vi "HOST_timesharelargearraywithdatacollection_2-27-23.vi"() -> ()   [LabVIEW 2020]
uses:
  <vilib>/rvi/interface/nirviMethod/nirviMethod.xnode
  <vilib>/rvi/errors/niLvFpgaMergeErrorWithErrorCode.vi
  <instrlib>/_niInstr/Streaming/v1/Host/niInstr Streaming v1 Host.lvlib
  <vilib>/rvi/interface/nirviReadWriteControl/nirviReadWriteControl.xnode
  <vilib>/rvi/interface/nirviCloseFPGA/nirviCloseFPGA.xnode
  <vilib>/rvi/interface/nirviOpenFPGA/nirviOpenFPGA.xnode
  <vilib>/rvi/interface/Simulation/niFpgaSimulationCallBeginRW.vi
  <vilib>/rvi/errors/niLvFpgaAdjustHostInterfaceError.vi
  NiFpgaLv.dll
  <vilib>/Utility/error.llb/Error Cluster From Error Code.vi
  <vilib>/Utility/file.llb/Write Delimited Spreadsheet (string).vi
  FPGA Bitfiles/rfsignal_FPGATarget_timesharelargear_57WzZEcFPMM.lvbitx
  <vilib>/FPGAPlugInAG/PXIe-7972R/niLvFpga_Open_PXIe-7972R.vi
  <vilib>/rvi/interface/common/dynamic/niFpgaDynamicAddResources.vi
  <vilib>/FPGAPlugInAG/Dynamic/niLvFpga_ConfigureFifo_Dynamic.vi
  <vilib>/FPGAPlugInAG/Dynamic/niLvFpga_StartFifo_Dynamic.vi
  <vilib>/FPGAPlugInAG/Dynamic/niLvFpga_WriteFifo_Dynamic.vi
  <vilib>/FPGAPlugInAG/Dynamic/niLvFpga_Close_Dynamic.vi
  <instrlib>/_niInstr/Streaming/v1/Host/Public/Start Continuous Stream.vi
  <instrlib>/_niInstr/Streaming/v1/Host/Public/Wait for Stream.vi
  <instrlib>/_niInstr/Streaming/v1/Host/Public/Start Finite Stream.vi
  <vilib>/FPGAPlugInAG/Dynamic/niLvFpga_ReadFifo_Dynamic.vi
  <vilib>/userDefined/Silver/nirio_resource_slv.ctl
  Controls/Clock Select.ctl
panel:
  in  "Data Trigger Level (V)":dbl
  in  "Record Size":u16=1024
  out "AI":waveform(dbl)[](graph)
  in  "Data Trigger When":enum8{"Trigger Above", "Trigger Below"}(ring)
  in  "Trigger Type":enum8{"Immediate", "Data Trigger", "TRIG input"}(ring)
  in  "Burst Power":bool
  in  "Correct Gains":bool
  in  "% of max CH 0":dbl=100.0
  in  "% of max CH 1":dbl=100.0
  in  "CH 1 Number of Waves":i8=1
  in  "write time ch0":bool
  in  "Record time for power sweep CH0":bool
  in  "Record time for power sweep CH1":bool
  in  "write time ch1":bool
  in  "save path for power calibration (dialog if empty)":path=path "D:/Lab Data/20220720/frequencysweep/CH0sweep-5to5.txt"
  out "time check":u16=1
  in  "Cycles per step":u16=30
  in  "Gain Scan Endpoint (CH1)":dbl[](array[numeric])=[0.0, 100.0, 100.0, 100.0, 100.0, 100.0, 100.0, 100.0, 100.0, 100.0]
  in  "Gain Scan Endpoint (CH0)":dbl[](array[numeric])=[100.0, 100.0, 100.0, 100.0, 100.0, 100.0, 100.0, 100.0, 100.0, 100.0, 100.0, 100.0, 100.0, 100.0, 100.0, 100.0, 100.0, 100.0, 100.0, 100.0, 100.0, 100.0, 100.0, 100.0, 100.0, 100.0, 100.0, 100.0, 100.0, 100.0, 100.0]
  in  "Scan End Setpoint (CH1)":dbl[](array[numeric])=[0.0, 1.0, 0.0, 0.0, 0.0, 0.0, 0.0, 0.0, 0.0, 0.0, 0.0, 0.0, 0.0, 0.0, 0.0, 0.0, 0.0, 0.0, 0.0, 0.0, 0.0, 0.0, 0.0, 0.0, 0.0, 0.0, 0.0, 0.0, 0.0, 0.0, 0.0] format="%#_10f"
  in  "Scan CH1":bool
  in  "Scan CH0":bool
  in  "Fq Scan Endpoint (CH0)":dbl[](array[numeric])=[0.0, 0.0, 0.0, 0.0, 0.0, 0.0, 0.0, 0.0, 0.0, 0.0, 0.0, 0.0, 0.0, 0.0, 0.0, 0.0, 0.0, 0.0, 0.0, 0.0, 0.0, 0.0, 0.0, 0.0, 0.0, 0.0, 0.0, 0.0, 0.0, 0.0, 0.0, 0.0, 0.0, 0.0, 0.0] format="%#_10f"
  in  "Amp mod on/off":bool[](array[boolean])=[FALSE, FALSE, FALSE, FALSE, FALSE, FALSE, FALSE, FALSE, FALSE, FALSE]
  in  "Mod Amp (%)":fxp<+,16,1>[](array[numeric])=[1.0, 1.0, 1.0, 1.0, 1.0, 1.0, 1.0, 1.0, 1.0, 1.0]
  in  "Mod Fq (Hz) 3":dbl[](array[numeric])=[1.0, 1.0, 1.0, 1.0, 1.0, 1.0, 1.0, 1.0, 1.0, 1.0] format="%#5.5f"
  in  "Wave 2 mod on/off":bool[](array[boolean])=[FALSE, FALSE, FALSE, FALSE, FALSE, FALSE, FALSE, FALSE, FALSE, FALSE]
  in  "Mod strength (Hz) 2":dbl[](array[numeric])=[100000.0, 100000.0, 100000.0, 100000.0, 100000.0, 100000.0, 100000.0, 100000.0, 100000.0, 100000.0] format="%#_6p"
  in  "Mod Fq (Hz) 2":dbl[](array[numeric])=[1.0, 1.0, 1.0, 1.0, 1.0, 1.0, 1.0, 1.0, 1.0, 1.0] format="%#5.5f"
  in  "Wave 1 mod on/off":bool[](array[boolean])=[FALSE, FALSE, FALSE, FALSE, FALSE, FALSE, FALSE, FALSE, FALSE, FALSE]
  in  "Mod strength (Hz)":dbl[](array[numeric])=[100000.0, 100000.0, 100000.0, 100000.0, 100000.0, 100000.0, 100000.0, 100000.0, 100000.0, 100000.0] format="%#_6p"
  in  "Mod Time (Hz)":dbl[](array[numeric])=[1.0, 1.0, 1.0, 1.0, 1.0, 1.0, 1.0, 1.0, 1.0, 1.0] format="%#5.5p"
  in  "Gain Scan Step Size % (CH1)":dbl=0.5
  in  "Gain Scan Step Size % (CH0)":dbl=0.1
  in  "Fq Scan Step Size MHz (CH1)":dbl=0.09999999999999999
  in  "Fq Scan Step Size MHz (CH0)":dbl=0.09999999999999999
  in  "CH 0 Number of Waves":i8=1
  in  "Wave Reader CH 1 (X)":dbl[](array[numeric])=[0.0, 1.0, 0.0, 0.0, 0.0, 0.0, 0.0, 0.0, 0.0, 0.0, 0.0, 0.0, 0.0, 0.0, 0.0, 0.0, 0.0, 0.0, 0.0, 0.0, 0.0, 0.0, 0.0, 0.0, 0.0, 0.0, 0.0, 0.0, 0.0, 0.0, 0.0] format="%#_15f"
  in  "Gain CH 1 (%)":dbl[](array[numeric])=[100.0, 0.0, 0.0, 0.0, 0.0, 0.0, 0.0, 0.0, 0.0, 0.0]
  in  "Remove transition edges":i32=5
  in  "Time per beam in us":i32=20
  in  "stop":bool
  in  "Gain CH 0 (%)":dbl[](array[numeric])=[100.0, 100.0, 100.0, 100.0, 100.0, 100.0, 100.0, 100.0, 100.0, 100.0, 100.0, 100.0, 100.0, 100.0, 100.0, 100.0, 100.0, 100.0, 100.0, 100.0, 100.0, 100.0, 100.0, 100.0, 100.0, 100.0, 100.0, 100.0, 100.0, 100.0, 100.0]
  in  "Wave Reader CH 0 (MHz from center)":dbl[](array[numeric])=[0.0, 0.0, 0.0, 0.0, 0.0, 0.0, 0.0, 0.0, 0.0, 0.0, 0.0, 0.0, 0.0, 0.0, 0.0, 0.0, 0.0, 0.0, 0.0, 0.0, 0.0, 0.0, 0.0, 0.0, 0.0, 0.0, 0.0, 0.0, 0.0, 0.0, 0.0, 0.0, 0.0, 0.0, 0.0] format="%#_13f"
  in  "Magnitude Initialization Vpp":dbl[](array[numeric])=[1.0, 1.0] format="%0.2p"
  in  "Frequencies (Hz)":dbl[](array[numeric])=[10000.0, 10000.0] format="%5.0p"
  in  "Signal Type":T1(ring)
  in  "Sampling Info":cluster{"Fs":dbl, "#s":dbl}={"Fs"=163840000.0, "#s"=65536.0} {"Fs" format="%#_5p"}
  out "Error Out":errorcluster
  in  "Update Waveform":bool
  in  "AO Channel":T2(ring)
  in  "Clock Select":T3 items=["Internal Clock", "Internal Clock w/ Ref via CLK/REF IN", "Internal Clock w/ Ref via Sync Clock", "External Clock via CLK/REF IN"]
  in  "Rate of External Sample Clock (MHz)":u16=100 min=60 max=100 step=1
  in  "RIO Resource":T4="RIO1"
  # "General Feedback Settings"
  # "Time cycle loop processing"
  # "Shared Feedback Controls"
  # "Don't change"
  # "Modulates the output frequencies of CH 1 in a sine wave pattern\n\nMod time: Sets how fast the modulation goes\n     (e.g. 1 Hz means it will go through a full cycle in 1 second)\n\nMod strength: Sets the amplitude of the modulation\n     (e.g. 100kHz means that the frequency will go between \n      set frequency + 100kHz and set frequency - 100kHz)"
  # "Modulates the output frequencies of CH 0 in a sine wave pattern\n\nMod time: Sets how fast the modulation goes\n     (e.g. 1 Hz means it will go through a full cycle in 1 second)\n\nMod strength: Sets the amplitude of the modulation\n     (e.g. 100kHz means that the frequency will go between \n      set frequency + 100kHz and set frequency - 100kHz)"
  # "Modulates the output amplitude of CH 0 in a sine wave pattern\n\nMod time: Sets how fast the modulation goes\n     (e.g. 1 Hz means it will go through a full cycle in 1 second)\n\nMod strength: Sets the amplitude of the modulation\n     (e.g. 5% means that the amplitude will go between \n      set amp + 5%  and set amp  - 5%)"
  # "Waveform Initialization"
  # "These allow you to smoothly ramp between frequencies or gain settings for each individual beam.\nThe channels scan independently, but it will simultaneously ramp every fq/gain in the channel to their desired point.\nThey should update to match the main control setting when scanning is not enabled."
  # "DO NOT CHANGE"
  # "Main control for the tones played on FPGA analog out 0\nSets the base, static frequency to play\n\nIt will play the first n rows of tones, \nwhere n is the \"# of beams\" value."
  # "Main control for the tones played on FPGA analog out 1\nSets the base, static frequency to play"
  # "Do not change these values while waiting for scan"
  # "Ch 0 Wave Sin Modulation"
  # "Ch 1 Wave Sin Modulation"
  # "Amplitude Sin Modulation"
  # "Ch 0 Output Waveforms"
  # "Ch 1 Output Waveforms"
  # "Ch0"
  # "Ch1"
  # "Controls the Output of the FPGA\nEach row corresponds to one beam created by the AOD\nCH 0 is Output 0 on the FPGA card and controls the () direction on the AOD; CH 1 is Output 1 on the FPGA card and controls the () direction on the AOD\n\n0 means that the center frequency (27MHz) is output. The total range is +-8MHz, but there too much efficiency loss after 4 MHz away from the center frequency\n\nThe gain is the percentage of the 1Vpp initialized voltage to output. It is in percentage and goes from 0 - 100"
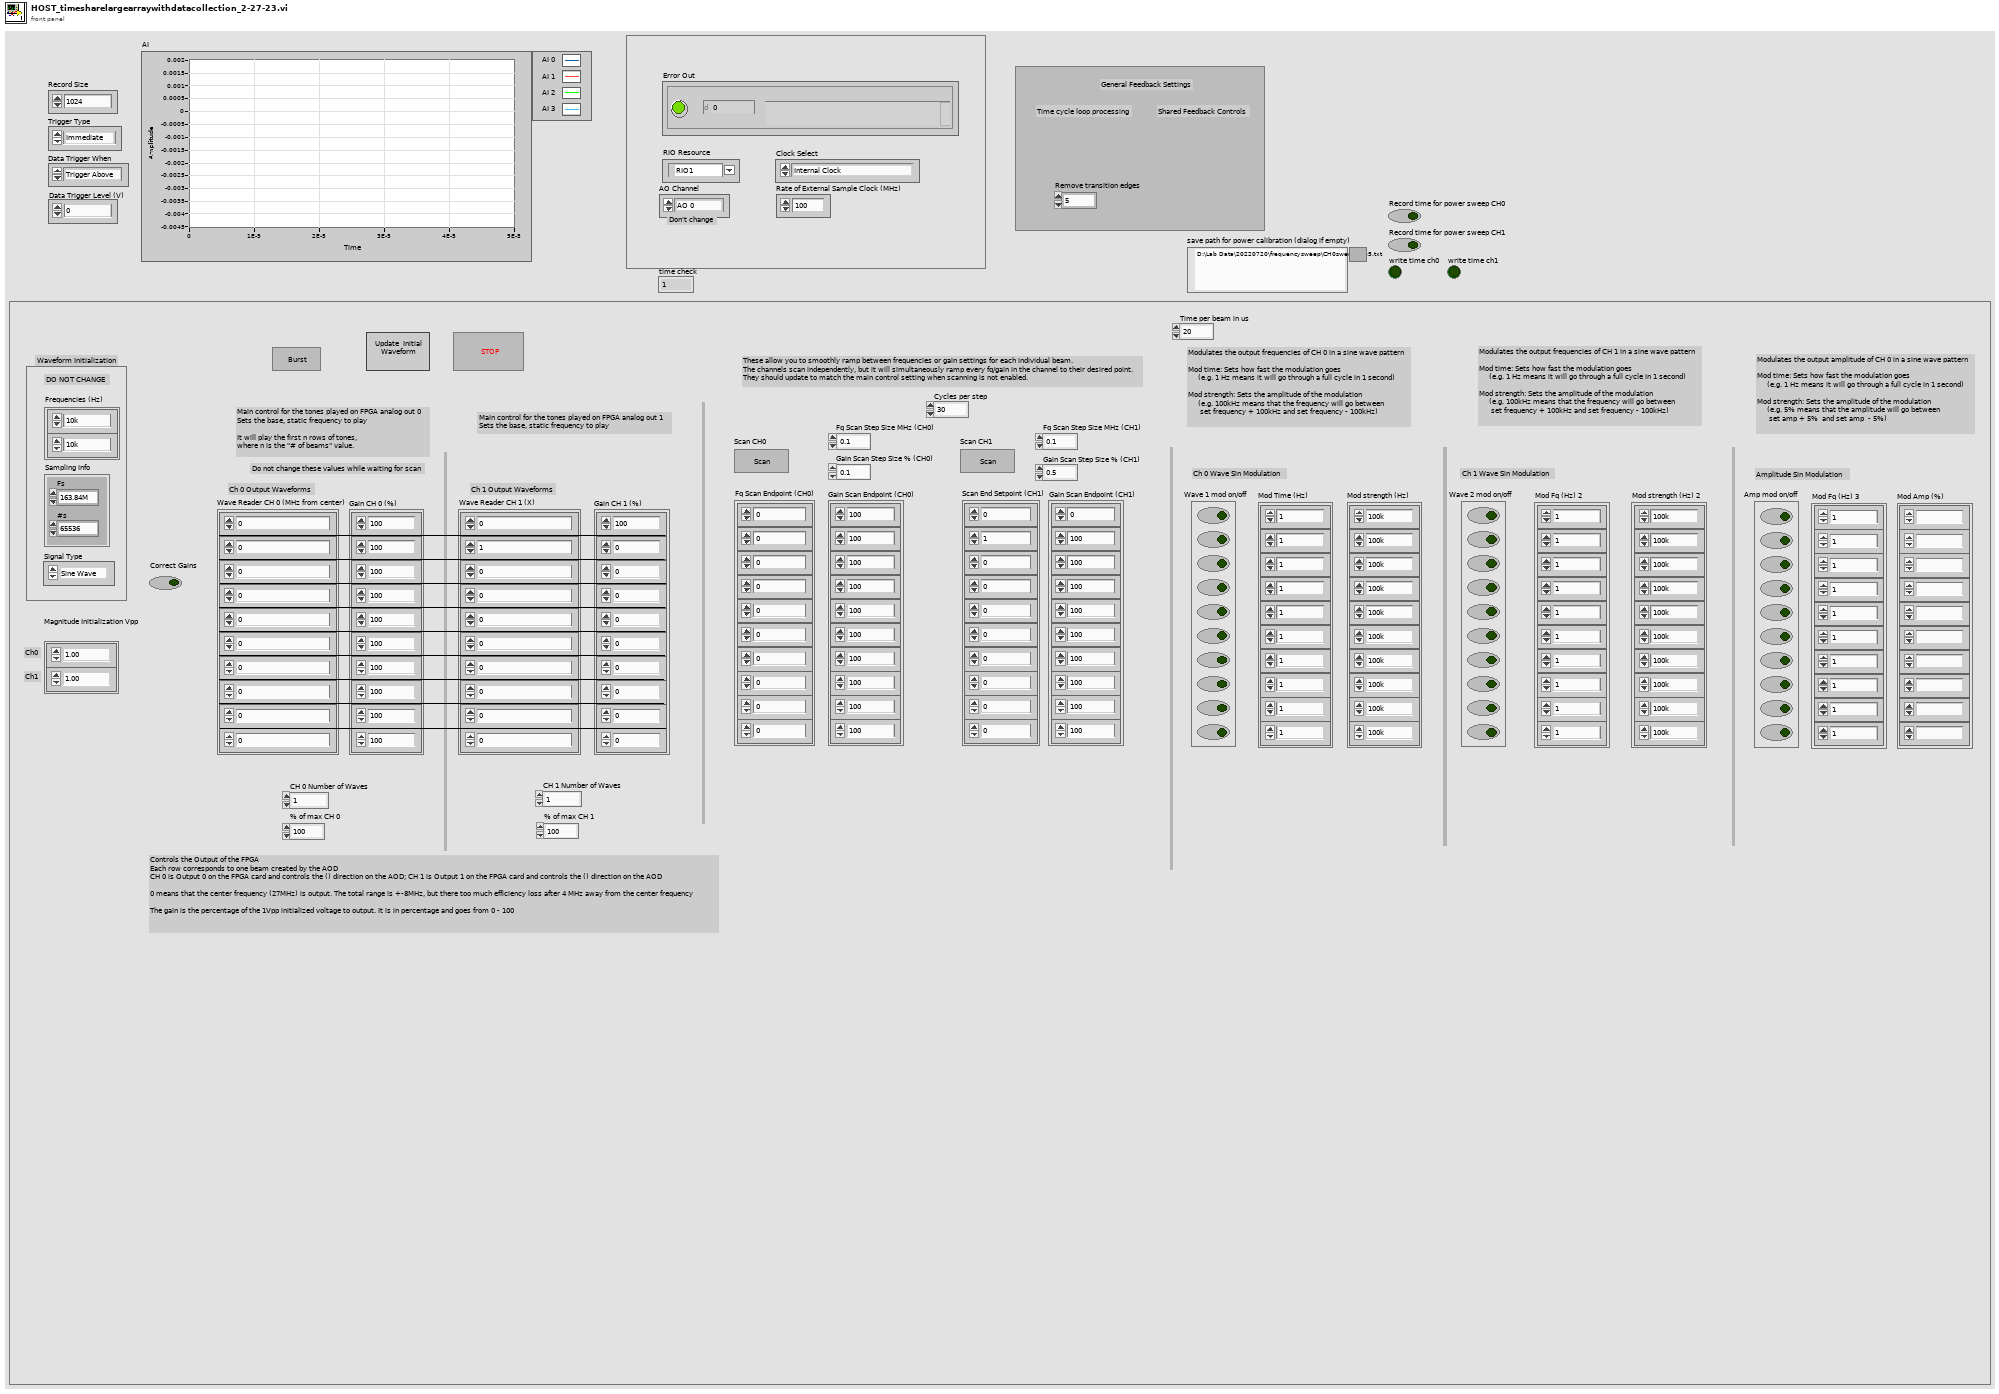
[diagram p1: front panel]
types:
  T1 = enum16{"Sine Wave", "Triangle Wave", "Square Wave", "Sawtooth Wave"}
  T2 = enum8{"AO 0", "AO 1", "AO 2", "AO 3", "AO 0, AO 1, AO 2, AO 3", "None"}
  T3 = typedef "Clock Select.ctl" = u16
  T4 = typedef "nirio_resource_slv.ctl" = tag
  T5 = cluster{"level":i16, "trigger when":enum8{"Trigger Above", "Trigger Below"}}
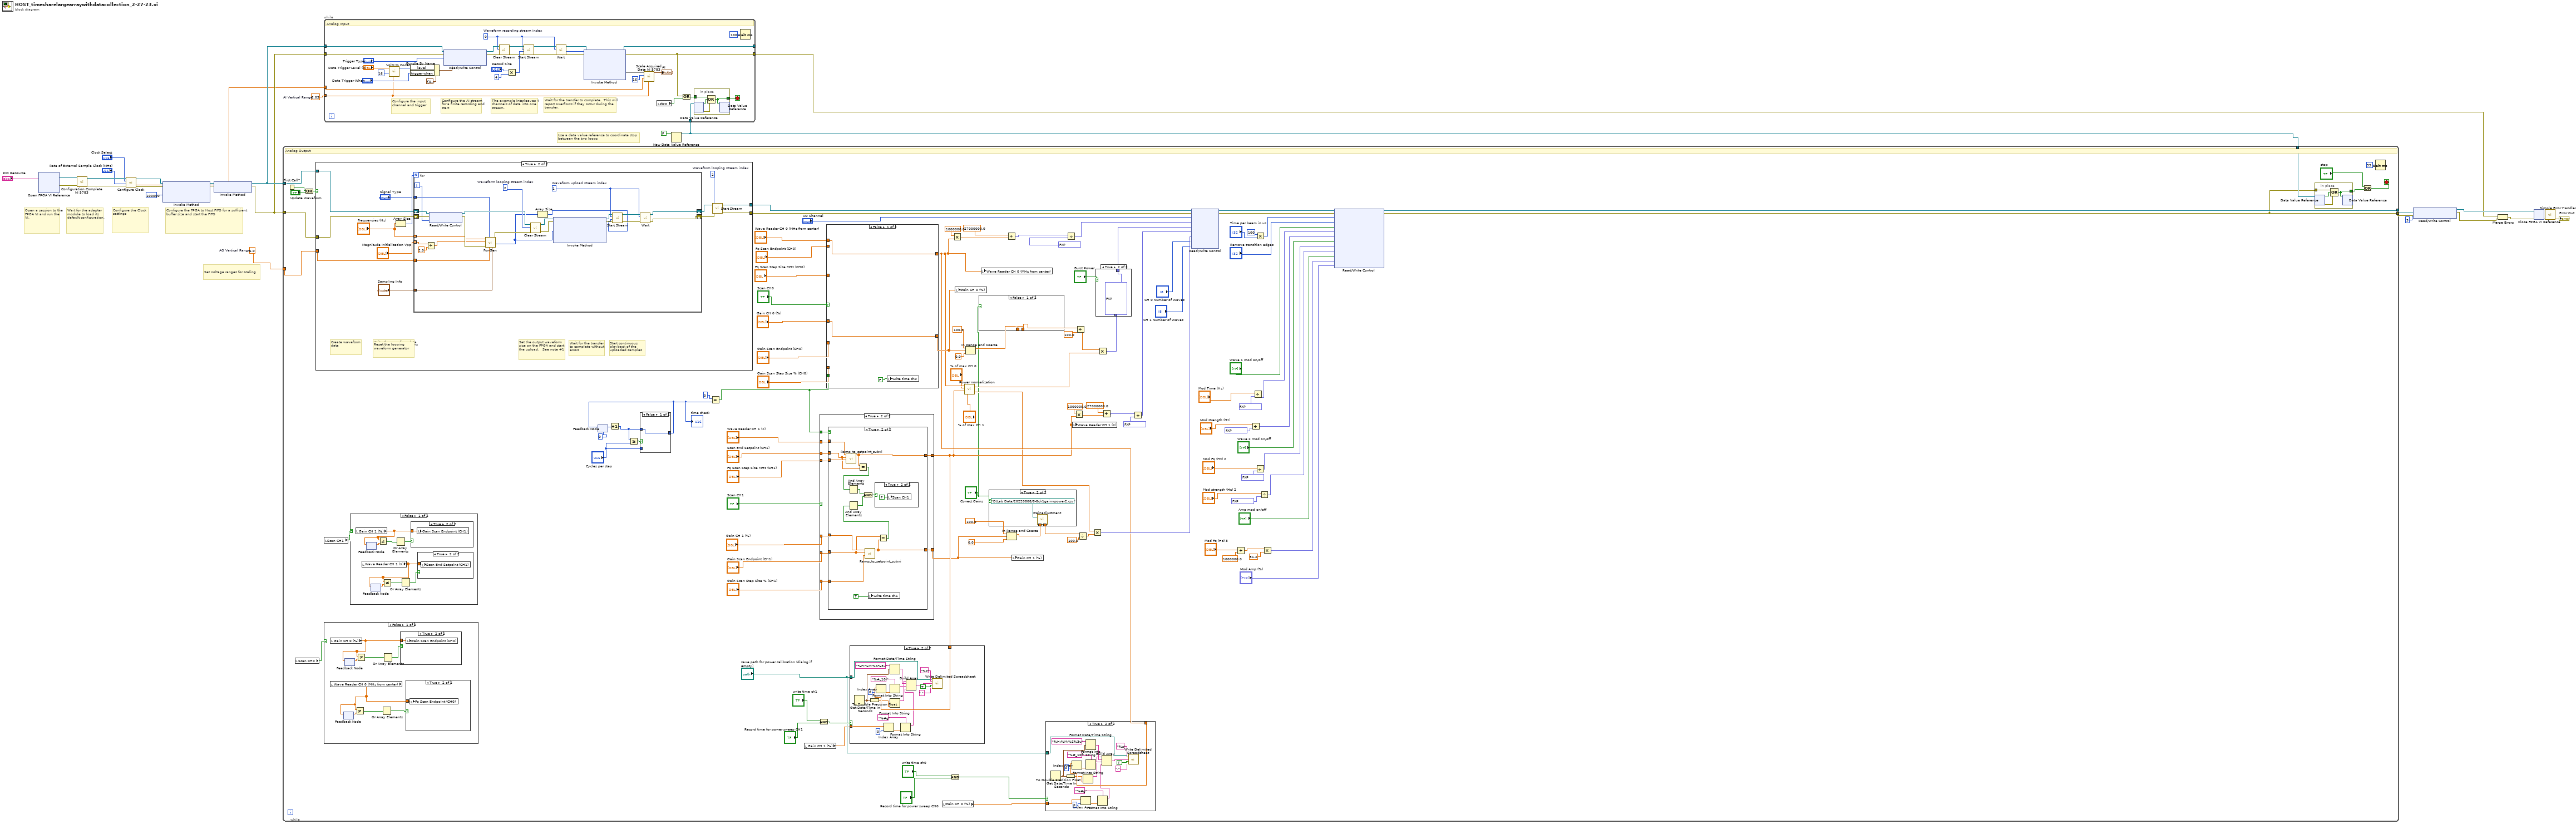
[diagram p0: block diagram]
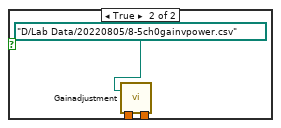
[diagram p3: hidden frame]
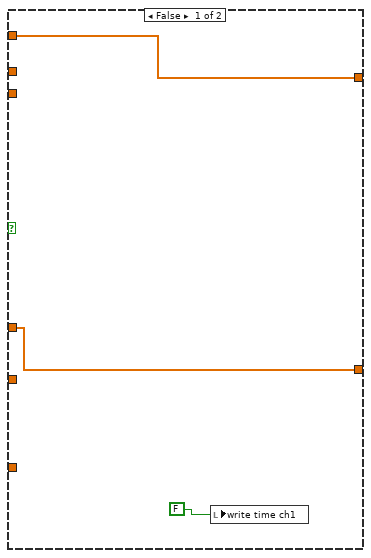
[diagram p7: hidden frame]
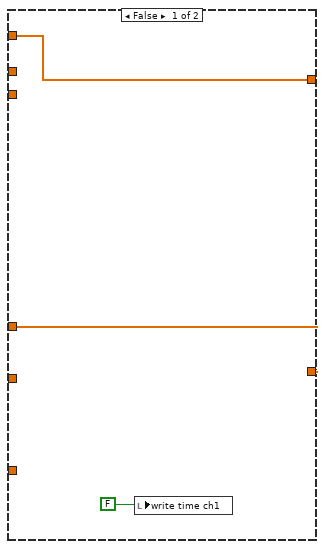
[diagram p8: hidden frame]
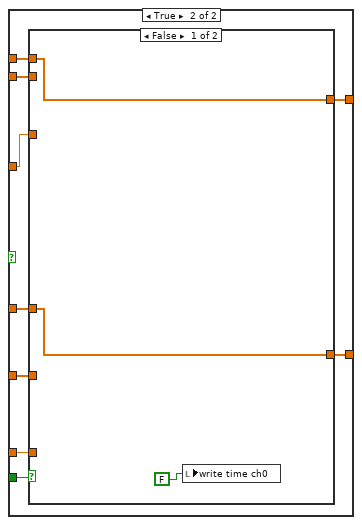
[diagram p10: hidden frame]
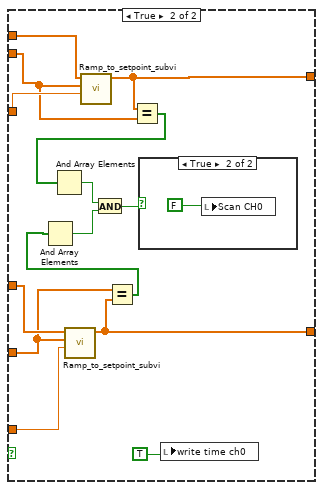
[diagram p11: hidden frame]
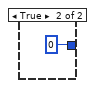
[diagram p13: hidden frame]
diagram:
  w4 = 2.03  # AI Vertical Range
  w16 = 1.0  # AO Vertical Range
  # "Use a data value reference to coordinate stop between the two loops"
  # "Set Voltage ranges for scaling"
  # "Configure the Clock settings"
  # "Configure the FPGA to Host FIFO for a sufficient buffer size and start the FIFO"
  # "Wait for the adapter module to load its default configuration."
  # "Open a session to the FPGA VI and run the VI."
  n1 = xnode "Open FPGA VI Reference"("resource name"="RIO Resource") -> ("FPGA VI Reference Out"=w14:refnum<k20>, "error out"=w13:errorcluster)  [unwired: 1 in]
  n2 = call "Configuration Complete NI 5783.vi"("error in"=w13, "FPGA VI Reference In"=w14) -> ("error out"=w24:errorcluster, "FPGA VI Reference Out"=w25:refnum<k20>)  [unwired: 7 in, 1 out]
  n3 = call "Configure Clock.vi"("error in (no error)"=w24, "Rate of External Sample Clock (MHz)"="Rate of External Sample Clock (MHz)", "Clock Select"="Clock Select", "FPGA VI Reference In"=w25) -> ("error out"=w22:errorcluster, "FPGA VI Reference Out"=w23:refnum<k20>, "Sampling Rate"=w5:dbl)  [unwired: 3 in, 2 out]
  n4 = xnode "Invoke Method"("FPGA VI Reference In"=w23, "error in"=w22, "Requested Depth"=u32 100000) -> ("FPGA VI Reference Out"=w28:refnum<k20>, "error out"=w27:errorcluster)  [unwired: 1 out]
  n5 = xnode "Invoke Method"("FPGA VI Reference In"=w28, "error in"=w27) -> ("FPGA VI Reference Out"=w7:refnum<k20>, "error out"=w6:errorcluster)
  n6 = New Data Value Reference(data value=FALSE ("Stopped")) -> (data value reference=w8:refnum<data-value>)  [unwired: 1 in, 1 out]
  n7 = while {
    tunnel: w6 -> [w137]
    tunnel: [w116] -> w12
    tunnel: w7 -> [w143]
    tunnel: [w117] -> w11
    tunnel: w8 -> [w138]
    tunnel: w16 -> [w136]
    stop <- w132 stop-if-true
    # "Analog Output"
    n8 = First Call?() -> (First Call?: T/F=w139:bool)
    n9 = local read "Scan CH0"() -> (w73:bool)
    n10 = Or(x=w139, y="Update Waveform") -> (x .or. y?=w140:bool)
    n11 = case shown="True" w140 {
      tunnel: [w281 w294] -> w135
      tunnel: [w280 w293] -> w134
      tunnel: w143 -> [w281 w291]
      tunnel: w137 -> [w280 w290]
      tunnel: w136 -> [_ w292]
      frame False {
      }
      frame True {
        w289 = 2  # Waveform looping stream index
        # "Loop over the waveforms to combine"
        # "Reset the looping waveform generator"
        # "Start continuous playback of the uploaded samples"
        # "Wait for the transfer to complete without errors"
        # "Set the output waveform size on the FPGA and start the upload.   See note #1"
        # "Write the waveform data to the FPGA for generation"
        # "Create waveform data"
        n12 = Array Size(array="Frequencies (Hz)") -> (size(s)=w284:i32)
        n13 = for {
          N: w284 -> [_]
          tunnel: w292 -> [w309]
          shift-right: [w303] -> w288
          shift-left: w291 -> [w308]
          shift-right: [w302] -> w287
          shift-left: w290 -> [w306]
          tunnel: "Frequencies (Hz)" -> [w301] mode=indexing
          tunnel: "Magnitude Initialization Vpp" -> [w297] mode=indexing
          tunnel: "Sampling Info" -> [w300]
          tunnel: "Signal Type" -> [w299]
          i -> [w298]
          w310 = 2  # Waveform looping stream index
          w315 = 1  # Waveform upload stream index
          n14 = Divide(x=w297, y=2.0) -> (x/y=w296:dbl)
          n15 = xnode "Read/Write Control"("FPGA VI Reference In"=w308, "error in"=w306, "Upload selector"=w298) -> ("FPGA VI Reference Out"=w307:refnum<k20>, "error out"=w305:errorcluster)
          n16 = call "FunGen.vi"("sampling info"=w300, "range (Vpp)"=w309, "signal type"=w299, "error in (no error)"=w305, "amplitude"=w296, "frequency"=w301) -> ("error out"=w311:errorcluster, "Waveform Data"=w304:i16[])  [unwired: 2 in, 2 out]
          n17 = call <instrlib>:"Clear Stream.vi"("error in (no error)"=w311, "stream index"=w310, "refnum in"=w307) -> ("error out"=w313:errorcluster, "refnum out"=w314:refnum<k20>)  [unwired: 7 in]
          n18 = Array Size(array=w304) -> (size(s)=w312:i32)
          n19 = xnode "Invoke Method"("FPGA VI Reference In"=w314, "error in"=w313, "Data"=w304) -> ("FPGA VI Reference Out"=w319:refnum<k20>, "error out"=w318:errorcluster)  [unwired: 1 in, 1 out]
          n20 = call-poly <instrlib>:"Start Stream.vi"("error in (no error)"=w318, "num samples"=w312, "stream index"=w315, "refnum in"=w319) -> ("error out"=w316:errorcluster, "refnum out"=w317:refnum<k20>)  [unwired: 6 in]
          n21 = call-poly <instrlib>:"Wait.vi"("error in (no error)"=w316, "stream index"=w315, "refnum in"=w317) -> ("error out"=w302:errorcluster, "refnum out"=w303:refnum<k20>)  [unwired: 5 in, 2 out]
        }
        n22 = call-poly <instrlib>:"Start Stream.vi"("error in (no error)"=w287, "stream index"=w289, "refnum in"=w288) -> ("error out"=w293:errorcluster, "refnum out"=w294:refnum<k20>)  [unwired: 7 in]
      }
    }
    n23 = local read "Scan CH1"() -> (w74:bool)
    n24 = case shown="False" w73 {
      frame False {
        n25 = local read "Gain CH 0 (%)"() -> (w256:dbl[])
        n26 = local read "Wave Reader CH 0 (MHz from center)"() -> (w263:dbl[])
        n27 = feedback-in #1(w263) -> ()
        n28 = feedback #1() -> (w262:dbl[])  [unwired: 1 in]
        n29 = feedback #2() -> (w259:dbl[])  [unwired: 1 in]
        n30 = feedback-in #2(w256) -> ()
        n31 = Not Equal?(x=w263, y=w262) -> (x != y?=w261:bool[])
        n32 = Not Equal?(x=w256, y=w259) -> (x != y?=w258:bool[])
        n33 = Or Array Elements(Boolean array=w261) -> (logical OR=w260:bool)
        n34 = Or Array Elements(Boolean array=w258) -> (logical OR=w257:bool)
        n35 = case shown="True" w257 {
          tunnel: w256 -> [_ w264]
          frame False {
          }
          frame True {
            n36 = local write "Gain Scan Endpoint (CH0)"(w264) -> ()
          }
        }
        n37 = case shown="True" w260 {
          tunnel: w263 -> [_ w265]
          frame False {
          }
          frame True {
            n38 = local write "Fq Scan Endpoint (CH0)"(w265) -> ()
          }
        }
      }
      frame True {
      }
    }
    n39 = case shown="False" w74 {
      frame False {
        n40 = local read "Gain CH 1 (%)"() -> (w266:dbl[])
        n41 = local read "Wave Reader CH 1 (X)"() -> (w270:dbl[])
        n42 = feedback #3() -> (w269:dbl[])  [unwired: 1 in]
        n43 = feedback-in #3(w266) -> ()
        n44 = feedback #4() -> (w273:dbl[])  [unwired: 1 in]
        n45 = feedback-in #4(w270) -> ()
        n46 = Not Equal?(x=w266, y=w269) -> (x != y?=w268:bool[])
        n47 = Not Equal?(x=w270, y=w273) -> (x != y?=w272:bool[])
        n48 = Or Array Elements(Boolean array=w268) -> (logical OR=w267:bool)
        n49 = Or Array Elements(Boolean array=w272) -> (logical OR=w271:bool)
        n50 = case shown="True" w267 {
          tunnel: w266 -> [_ w274]
          frame False {
          }
          frame True {
            n51 = local write "Gain Scan Endpoint (CH1)"(w274) -> ()
          }
        }
        n52 = case shown="True" w271 {
          tunnel: w270 -> [_ w275]
          frame False {
          }
          frame True {
            n53 = local write "Scan End Setpoint (CH1)"(w275) -> ()
          }
        }
      }
      frame True {
      }
    }
    n54 = feedback #5(u16 0) -> (w69:u16)
    n55 = Increment(x=w69) -> (x+1=w67:u16)
    n56 = Greater Or Equal?(x=w67, y="Cycles per step") -> (x >= y?=w68:bool)
    n57 = case shown="False" w68 {
      tunnel: w67 -> [w254 _]
      tunnel: "Cycles per step" -> [_ _]
      tunnel: [w254 u16 0] -> w61
      frame False {
      }
      frame True {
      }
    }
    "time check" <- w61
    n58 = feedback-in #5(w61) -> ()
    n59 = Equal?(x=u16 0, y=w61) -> (x = y?=w63:bool)
    n60 = local read "Gain CH 1 (%)"() -> (w37:dbl[])
    n61 = And(x="write time ch1", y="Record time for power sweep CH1") -> (x .and. y?=w60:bool)
    n62 = case shown="True" "Scan CH1" {
      tunnel: "Fq Scan Step Size MHz (CH1)" -> [_ w205]
      tunnel: [w196 w204] -> w50
      tunnel: "Wave Reader CH 1 (X)" -> [w196 w203]
      tunnel: "Scan End Setpoint (CH1)" -> [_ w202]
      tunnel: "Gain Scan Step Size % (CH1)" -> [_ w201]
      tunnel: "Gain CH 1 (%)" -> [w195 w200]
      tunnel: "Gain Scan Endpoint (CH1)" -> [_ w199]
      tunnel: [w195 w198] -> w39
      tunnel: w63 -> [_ w197]
      frame False {
        n63 = local write "write time ch1"(FALSE) -> ()
      }
      frame True {
        n64 = case shown="True" w197 {
          tunnel: w203 -> [w208 w222]
          tunnel: w202 -> [_ w220]
          tunnel: w205 -> [_ w221]
          tunnel: [w208 w219] -> w204
          tunnel: w200 -> [w207 w217]
          tunnel: w199 -> [_ w216]
          tunnel: w201 -> [_ w215]
          tunnel: [w207 w210] -> w198
          frame False {
            n65 = local write "write time ch1"(FALSE) -> ()
          }
          frame True {
            n66 = call "Ramp_to_setpoint_subvi.vi"("Numeric"=w221, "Scan to Fq (CH0)"=w220, "Wave Reader CH 0 (Y)"=w222) -> ("Array"=w219:dbl[])  [unwired: 8 in]
            n67 = Equal?(x=w219, y=w220) -> (x = y?=w218:bool[])
            n68 = And Array Elements(Boolean array=w218) -> (logical AND=w212:bool)
            n69 = call "Ramp_to_setpoint_subvi.vi"("Numeric"=w215, "Scan to Fq (CH0)"=w216, "Wave Reader CH 0 (Y)"=w217) -> ("Array"=w210:dbl[])  [unwired: 8 in]
            n70 = local write "write time ch1"(TRUE) -> ()
            n71 = Equal?(x=w216, y=w210) -> (x = y?=w211:bool[])
            n72 = And Array Elements(Boolean array=w211) -> (logical AND=w213:bool)
            n73 = And(x=w212, y=w213) -> (x .and. y?=w214:bool)
            n74 = case shown="True" w214 {
              frame False {
              }
              frame True {
                n75 = local write "Scan CH1"(FALSE) -> ()
              }
            }
          }
        }
      }
    }
    n76 = case shown="False" "Scan CH0" {
      tunnel: "Fq Scan Step Size MHz (CH0)" -> [_ w235]
      tunnel: "Wave Reader CH 0 (MHz from center)" -> [w226 w234]
      tunnel: "Fq Scan Endpoint (CH0)" -> [_ w233]
      tunnel: [w226 w232] -> w51
      tunnel: "Gain CH 0 (%)" -> [w225 w231]
      tunnel: "Gain Scan Endpoint (CH0)" -> [_ w230]
      tunnel: [w225 w229] -> w78
      tunnel: "Gain Scan Step Size % (CH0)" -> [_ w228]
      tunnel: w63 -> [_ w227]
      frame False {
        n77 = local write "write time ch0"(FALSE) -> ()
      }
      frame True {
        n78 = case shown="False" w227 {
          tunnel: w234 -> [w238 w252]
          tunnel: w233 -> [_ w250]
          tunnel: w235 -> [_ w251]
          tunnel: [w238 w249] -> w232
          tunnel: w231 -> [w237 w247]
          tunnel: w230 -> [_ w244]
          tunnel: w228 -> [_ w246]
          tunnel: [w237 w245] -> w229
          frame False {
            n79 = local write "write time ch0"(FALSE) -> ()
          }
          frame True {
            n80 = call "Ramp_to_setpoint_subvi.vi"("Numeric"=w246, "Scan to Fq (CH0)"=w244, "Wave Reader CH 0 (Y)"=w247) -> ("Array"=w245:dbl[])  [unwired: 8 in]
            n81 = call "Ramp_to_setpoint_subvi.vi"("Numeric"=w251, "Scan to Fq (CH0)"=w250, "Wave Reader CH 0 (Y)"=w252) -> ("Array"=w249:dbl[])  [unwired: 8 in]
            n82 = Equal?(x=w244, y=w245) -> (x = y?=w243:bool[])
            n83 = And Array Elements(Boolean array=w243) -> (logical AND=w240:bool)
            n84 = Equal?(x=w249, y=w250) -> (x = y?=w248:bool[])
            n85 = And Array Elements(Boolean array=w248) -> (logical AND=w241:bool)
            n86 = And(x=w241, y=w240) -> (x .and. y?=w242:bool)
            n87 = case shown="True" w242 {
              frame False {
              }
              frame True {
                n88 = local write "Scan CH0"(FALSE) -> ()
              }
            }
            n89 = local write "write time ch0"(TRUE) -> ()
          }
        }
      }
    }
    n90 = case shown="True" w60 {
      tunnel: w50 -> [_ w186]
      tunnel: "save path for power calibration (dialog if empty)" -> [_ w179]
      tunnel: w37 -> [_ w174]
      frame False {
      }
      frame True {
        n91 = Get Date/Time In Seconds() -> (seconds since 1Jan1904=w182:timestamp)
        n92 = To Double Precision Float(number=w182) -> (double precision float=w181:dbl)
        n93 = Index Array(array=w186, index=0) -> (element=w184:dbl)
        n94 = Index Array(array=w174, index=0) -> (element=w177:dbl)
        n95 = Format Date/Time String(time format string (%c)="%H:%M:%S%3u", seconds (now)=w182) -> (date/time string=w189:string)  [unwired: 1 in]
        n96 = Format Into String(format string="%#_10f", w184) -> (resulting string=w188:string)  [unwired: 2 in, 1 out]
        n97 = Format Into String(w181) -> (resulting string=w180:string)  [unwired: 3 in, 1 out]
        n98 = Format Into String(format string="%#g", w177) -> (resulting string=w176:string)  [unwired: 2 in, 1 out]
        n99 = Build Array(w180, w189, w188, w176) -> (w183:string[])
        n100 = call-poly <vilib>:"Write Delimited Spreadsheet.vi"("file path (dialog if empty)"=w179, "format (%s)"="%s" ("format (%.3f)"), "1D data"=w183, "append to file? (new file:F)"=TRUE, "delimiter (\\t)"="," ("delimiter (\\t)")) -> ()  [unwired: 9 in, 2 out]
      }
    }
    n101 = local read "Gain CH 0 (%)"() -> (w38:dbl[])
    n102 = And(x="write time ch0", y="Record time for power sweep CH0") -> (x .and. y?=w56:bool)
    n103 = Multiply(x=1000000.0, y=w51) -> (x*y=w94:dbl[])
    n104 = local write "Gain CH 0 (%)"(w78) -> ()
    n105 = call "Power normalization.vi"("% of max CH 1"="% of max CH 1", "CH 1 frequency"=w50, "% of max CH 0"="% of max CH 0", "CH 0 frequency"=w51) -> ("Normalized CH1"=w40:dbl[], "Normalized CH 0"=w49:dbl[])
    n106 = In Range and Coerce(upper limit=100.0, x=w78, lower limit=0.0) -> (coerced(x)=w36:dbl[])  [unwired: 1 out]
    n107 = case shown="False" "Correct Gains" {
      tunnel: w36 -> [w146 w149]
      tunnel: [w146 w148] -> w35
      frame False {
      }
      frame True {
        n108 = call "Gainadjustment.vi"("Gain"=w149, "CH 0 Data Path (.csv)"=path "D:/Lab Data/20220805/8-5ch0gainvpower.csv" ("CH0 Gain correction path")) -> ("Adjusted gain"=w148:dbl[])
      }
    }
    n109 = local write "Wave Reader CH 0 (MHz from center)"(w51) -> ()
    n110 = Add(x=27000000.0, y=w94) -> (x+y=w91:fxp<+/-,64,32>[])
    n111 = In Range and Coerce(upper limit=100.0, x=w39, lower limit=0.0) -> (coerced(x)=w34:dbl[])  [unwired: 1 out]
    n112 = case shown="True" "Correct Gains" {
      tunnel: w34 -> [w150 w152]
      tunnel: [w150 w151] -> w33
      frame False {
      }
      frame True {
        n113 = call "Gainadjustment.vi"("Gain"=w152, "CH 0 Data Path (.csv)"=path "D:/Lab Data/20220808/8-8ch1gainvpower2.csv" ("CH0 Gain correction path")) -> ("Adjusted gain"=w151:dbl[])
      }
    }
    n114 = local write "Gain CH 1 (%)"(w39) -> ()
    n115 = case shown="True" w56 {
      tunnel: w51 -> [_ w166]
      tunnel: "save path for power calibration (dialog if empty)" -> [_ w159]
      tunnel: w38 -> [_ w154]
      frame False {
      }
      frame True {
        n116 = Get Date/Time In Seconds() -> (seconds since 1Jan1904=w162:timestamp)
        n117 = To Double Precision Float(number=w162) -> (double precision float=w161:dbl)
        n118 = Index Array(array=w166, index=0) -> (element=w164:dbl)
        n119 = Index Array(array=w154, index=0) -> (element=w157:dbl)
        n120 = Format Into String(w161) -> (resulting string=w160:string)  [unwired: 3 in, 1 out]
        n121 = Format Date/Time String(time format string (%c)="%H:%M:%S%3u", seconds (now)=w162) -> (date/time string=w169:string)  [unwired: 1 in]
        n122 = Format Into String(format string="%#_10f", w164) -> (resulting string=w168:string)  [unwired: 2 in, 1 out]
        n123 = Format Into String(format string="%#g", w157) -> (resulting string=w155:string)  [unwired: 2 in, 1 out]
        n124 = Build Array(w160, w169, w168, w155) -> (w163:string[])
        n125 = call-poly <vilib>:"Write Delimited Spreadsheet.vi"("file path (dialog if empty)"=w159, "format (%s)"="%s" ("format (%.3f)"), "1D data"=w163, "append to file? (new file:F)"=TRUE, "delimiter (\\t)"="," ("delimiter (\\t)")) -> ()  [unwired: 9 in, 2 out]
      }
    }
    n126 = Divide(x=w91, y=fxp<+,32,16> 6103.515625) -> (x/y=w123:fxp<+,33,16>[])
    n127 = local write "Wave Reader CH 1 (X)"(w50) -> ()
    n128 = Multiply(x=1000000.0, y=w50) -> (x*y=w88:dbl[])
    n129 = Divide(x=w35, y=100.0) -> (x/y=w44:dbl[])
    n130 = Divide(x=w33, y=100.0) -> (x/y=w41:dbl[])
    n131 = Multiply(x=w40, y=w41) -> (x*y=w62:fxp<+,32,5>[])
    n132 = Multiply(x=w44, y=w49) -> (x*y=w30:fxp<+,32,5>[])
    n133 = case shown="True" "Burst Power" {
      tunnel: [w144 fxp<+,32,5>[] [1.0, 1.0, 1.0, 1.0, 1.0, 1.0, 1.0, 1.0, 1.0, 1.0]] -> w31
      tunnel: w30 -> [w144 _]
      frame False {
      }
      frame True {
      }
    }
    n134 = Add(x=27000000.0, y=w88) -> (x+y=w85:fxp<+/-,64,32>[])
    n135 = Divide(x=w85, y=fxp<+,32,16> 6103.515625) -> (x/y=w121:fxp<+,33,16>[])
    n136 = xnode "Read/Write Control"("FPGA VI Reference In"=w135, "error in"=w134, "AO Channel"="AO Channel", "Wave 1 Set"=w123, "Amp Set 1"=w31, "Wave 2 Set"=w121, "Amp 2"=w62, "Ch 0 size"="CH 0 Number of Waves", "CH 1 Size"="CH 1 Number of Waves") -> ("FPGA VI Reference Out"=w128:refnum<k20>, "error out"=w127:errorcluster)
    n137 = Divide(x="Mod Fq (Hz) 3", y=1000000.0) -> (x/y=w113:dbl[])
    n138 = Divide(x="Mod strength (Hz)", y=fxp<+,32,16> 6103.515625) -> (x/y=w108:fxp<+,32,16>[])
    n139 = Divide(x="Mod Time (Hz)", y=fxp<+,32,16> 6103.515625) -> (x/y=w101:fxp<+,32,13>[])
    n140 = Divide(x="Mod Fq (Hz) 2", y=fxp<+,32,16> 6103.515625) -> (x/y=w98:fxp<+,32,13>[])
    n141 = Multiply(x=100, y="Time per beam in us") -> (x*y=w124:i32)
    n142 = Divide(x="Mod strength (Hz) 2", y=fxp<+,32,16> 6103.515625) -> (x/y=w106:fxp<+,32,16>[])
    n143 = Multiply(x=w113, y=51.2) -> (x*y=w104:fxp<+,32,13>[])
    n144 = xnode "Read/Write Control"("FPGA VI Reference In"=w128, "error in"=w127, "Timeshare"=w124, "Edge size"="Remove transition edges", "Wave 1 freq mod (on/off)"="Wave 1 mod on/off", "Wave 1 freq mod f"=w101, "Wave 1 freq mod gain"=w108, "Wave 2 freq mod (on/off)"="Wave 2 mod on/off", "Wave 2 freq mod f"=w98, "Wave 2 freq mod gain"=w106, "Amp mod (on/off)"="Amp mod on/off", "Amp mod f"=w104, "Amp mod gain"="Mod Amp (%)") -> ("FPGA VI Reference Out"=w117:refnum<k20>, "error out"=w116:errorcluster)
    n145 = in-place {
      in-place-border: [w277] -> w131
      in-place-border: w116 -> [w279]
      n146 = in-place-dvr #6(w138) -> (w278:bool, w276:errorcluster)
      n147 = Compound Arithmetic op=OR(w279, w278, w276) -> (w277:bool)
      n148 = in-place-dvr #6(w277) -> ()  [unwired: 2 out]
    }
    n149 = Or(x="stop", y=w131) -> (x .or. y?=w132:bool)
    n150 = Wait (ms)(milliseconds to wait=u32 33) -> ()  [unwired: 1 out]
  }
  n151 = while {
    tunnel: [w352] -> _
    tunnel: w7 -> [w351]
    tunnel: w4 -> [w330]
    tunnel: w8 -> [w348]
    tunnel: w6 -> [w350]
    tunnel: [w336] -> w1
    tunnel: w5 -> [w331]
    stop <- w349 stop-if-true
    w321 = 0  # Waveform recording stream index
    # "The example interleaves 4 channels of data into one stream."
    # "Wait for the transfer to complete.  This will report overflows if they occur during the transfer."
    # "Configure the AI stream for a finite recording and start"
    # "Configure the input channel and trigger"
    # "Analog Input"
    n152 = call "Volts to Codes.vi"("range (Vpp)"=w330, "Number of Bits"=i16 16, "Volts In"="Data Trigger Level (V)") -> ("ADC Codes Out"=w332:i16)  [unwired: 8 in]
    n153 = Bundle By Name(cluster=T5 {"level"=0, "trigger when"=enum."Trigger Above"} ("Trigger Configuration"), "level"=w332, "trigger when"="Data Trigger When") -> (w335:T5)
    n154 = xnode "Read/Write Control"("FPGA VI Reference In"=w351, "error in"=w350, "Trigger Type"="Trigger Type", "Trigger Configuration"=w335) -> ("FPGA VI Reference Out"=w325:refnum<k20>, "error out"=w324:errorcluster)
    n155 = call <instrlib>:"Clear Stream.vi"("error in (no error)"=w324, "stream index"=w321, "refnum in"=w325) -> ("error out"=w323:errorcluster, "refnum out"=w322:refnum<k20>)  [unwired: 7 in]
    n156 = Multiply(x="Record Size", y=u16 4) -> (x*y=w327:u16)
    n157 = call-poly <instrlib>:"Start Stream.vi"("error in (no error)"=w323, "num samples"=w327, "stream index"=w321, "refnum in"=w322) -> ("error out"=w341:errorcluster, "refnum out"=w339:refnum<k20>)  [unwired: 6 in]
    n158 = call-poly <instrlib>:"Wait.vi"("error in (no error)"=w341, "stream index"=w321, "refnum in"=w339) -> ("error out"=w337:errorcluster, "samples transferred"=w340:u64, "refnum out"=w338:refnum<k20>)  [unwired: 5 in, 1 out]
    n159 = xnode "Invoke Method"("FPGA VI Reference In"=w338, "error in"=w337, "Number of Elements"=w340) -> ("FPGA VI Reference Out"=w352:refnum<k20>, "error out"=w336:errorcluster, "Data"=w344:void[])  [unwired: 1 in, 1 out]
    n160 = call "Scale Acquired Data NI 5783.vi"("range (V)"=w330, "Sample Rate"=w331, "Number of Bits"=i16 16, "Data In"=w344) -> ("Data"=→"AI":waveform(dbl)[])  [unwired: 7 in]
    n161 = local read "stop"() -> (w320:bool)
    n162 = Or(x=w336, y=w320) -> (x .or. y?=w347:bool)
    n163 = in-place {
      in-place-border: [w355] -> w349
      in-place-border: w347 -> [w357]
      n164 = in-place-dvr #7(w348) -> (w356:bool, w354:errorcluster)
      n165 = Compound Arithmetic op=OR(w357, w356, w354) -> (w355:bool)
      n166 = in-place-dvr #7(w355) -> ()  [unwired: 2 out]
    }
    n167 = Wait (ms)(milliseconds to wait=u32 100) -> ()  [unwired: 1 out]
  }
  n168 = xnode "Read/Write Control"("FPGA VI Reference In"=w11, "error in"=w12, "stream.request state 2"=3) -> ("FPGA VI Reference Out"=w9:refnum<k20>, "error out"=w2:errorcluster)
  n169 = Merge Errors(w1, w2) -> (w3:errorcluster)
  n170 = xnode "Close FPGA VI Reference"("FPGA VI Reference In"=w9, "error in"=w3) -> ("error out"=w19:errorcluster)
  n171 = call <vilib>:"Simple Error Handler.vi"("error in (no error)"=w19) -> ("error out"=→"Error Out":errorcluster)  [unwired: 4 in, 4 out]
